vi "Write Helm Rate (Hz) Actor.vi"(8 "error in (no error)":errorcluster, 10 "Helm Rate (Hz)":dbl, 11 "RDS Helm Actor in":refnum<class "RDS Helm Actor.lvclass">) -> (0 "error out":errorcluster, 3 "RDS Helm Actor out":refnum<class "RDS Helm Actor.lvclass">)   [LabVIEW 2015, in "RDS Helm Actor.lvlib" / "RDS Helm Actor.lvclass"]
uses:
  RDS Helm Actor.lvclass
  RDS Helm Actor.lvclass/RDS Helm Actor.ctl
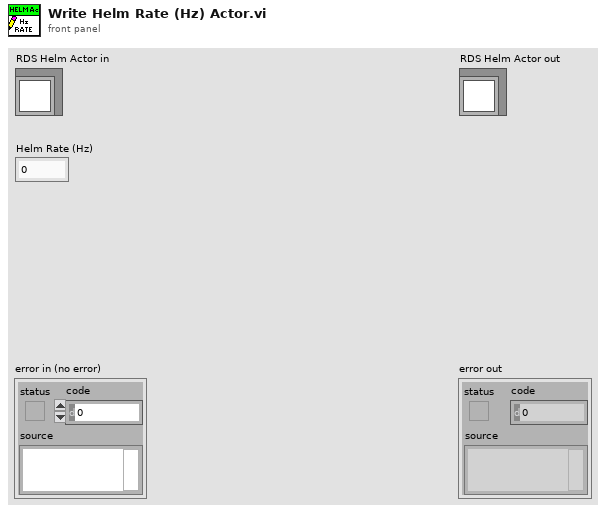
[diagram p1: front panel]
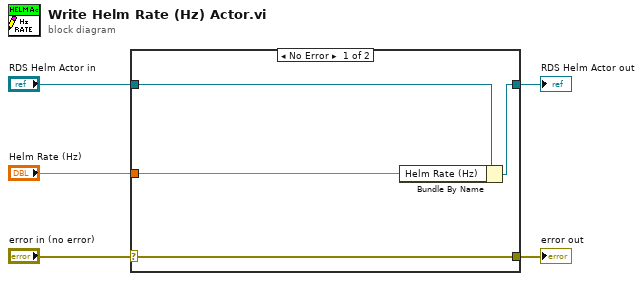
[diagram p0: block diagram]
diagram:
  n1 = case shown="No Error" "error in (no error)" {
    selector: "error in (no error)" -> [w9 w10]
    tunnel: [w9 w10] -> w4
    tunnel: [w7 w11] -> w2
    tunnel: "RDS Helm Actor in" -> [w8 w11]
    tunnel: "Helm Rate (Hz)" -> [w6 _]
    frame No Error {
      n2 = Bundle By Name(cluster=w8, "Helm Rate (Hz)"=w6) -> (w7:refnum<class "RDS Helm Actor.lvclass">)
    }
    frame Error {
    }
  }
  "error out" <- w4
  "RDS Helm Actor out" <- w2
